vi "GPS.vi"(0 "Data Requested":u16(ring) items=["Time (UTC)"=0, "Status"=1, "Latitude"=2, "Longitude"=4, "Velocity (cm/s)"=6, "Heading (degrees)"=7, "Dist to destination (m)"=8, "Angle to destination (degrees)"=9, "Angle since last req"=10, "Set Destination Latitude"=11, "Set Destination Longitude"=12], 2 "NXT":T1, 3 "Port":T2 items=["Port 1", "Port 2", "Port 3", "Port 4"]) -> (1 "value":i32 format="%.0x", 4 "NXT":T1)   [LabVIEW 2010]
uses:
  <vilib>/NXT/Subs/LVHSConnector.ctl
  <vilib>/NXT/Block Support/NXT_InputPort.ctl
  <vilib>/NXT/Block Support/HWPage.SensorType.ctl
  <vilib>/NXT/Block Support/HWPage.SensorMode.ctl
panel:
  out "Bytes read":u8[](array[numeric]) format="%.0x"
  # "¥ Latitude is represented by an 8-digit integer. If the position is in the northern hemisphere, the number is positive. If the position is in the southern hemisphere, the latitude is negative.\n¥ Longitude is represented by a 9-digit integer. If the position is in the eastern hemisphere, the longitude is positive. If the position is in the western hemisphere, the longitude is negative."
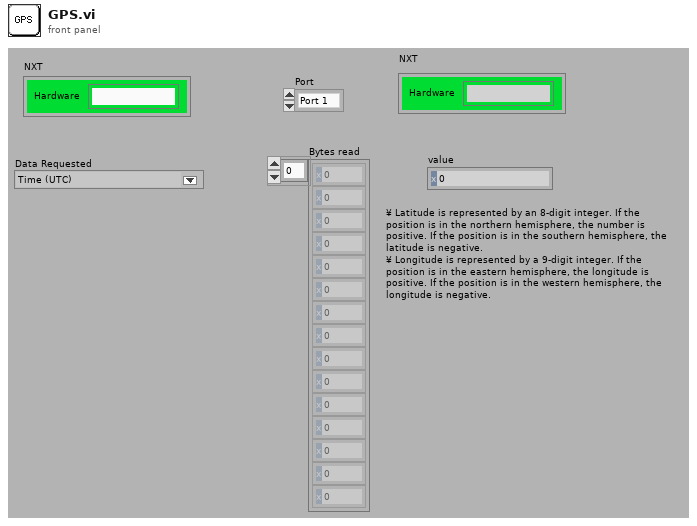
[diagram p1: front panel]
types:
  T1 = typedef "LVHSConnector.ctl" = cluster{"Hardware":string, "Flattened String":string}
  T2 = typedef "NXT_InputPort.ctl" = u8
  T3 = typedef "HWPage.SensorType.ctl" = u8
  T4 = typedef "HWPage.SensorMode.ctl" = u8
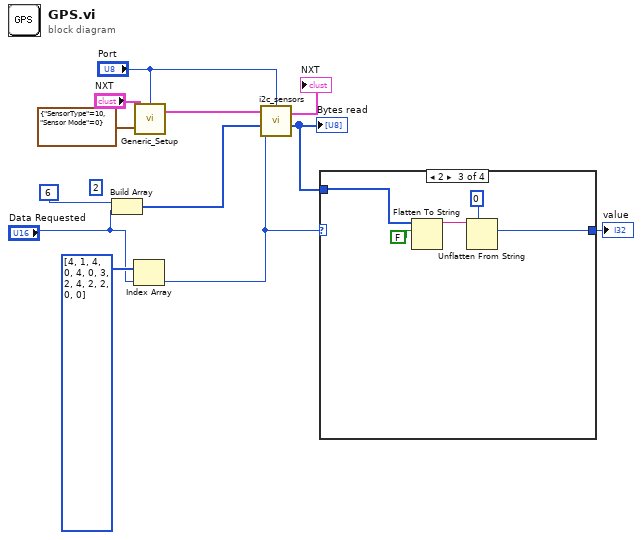
[diagram p0: block diagram]
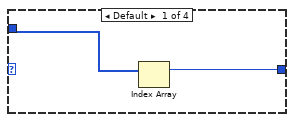
[diagram p2: hidden frame]
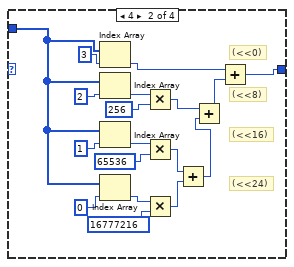
[diagram p3: hidden frame]
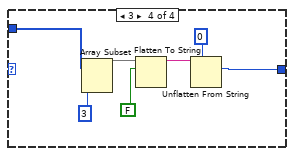
[diagram p4: hidden frame]
diagram:
  (unwired) u8 2 ("Return Length")
  n1 = Build Array(u8 6, "Data Requested") -> (w8:u16[])
  n2 = Index Array(array=u8[] [4, 1, 4, 0, 4, 0, 3, 2, 4, 2, 2, 0, 0], index="Data Requested") -> (element=w1:u8)
  n3 = call <vilib>:"Generic_Setup.vi"("Sensor Setup"=cluster{"SensorType":T3, "Sensor Mode":T4} {"SensorType"=10, "Sensor Mode"=0}, "NXT"="NXT", "Port"="Port") -> ("NXT"=w12:T1)  [unwired: 1 out]
  n4 = call <vilib>:"i2c_sensors.vi"("Return Length"=w1, "Bytes to Write"=w8, "NXT"=w12, "Port"="Port") -> ("Bytes read"=w2:u8[], "NXT"=→"NXT":T1)  [unwired: 1 in, 1 out]
  "Bytes read" <- w2
  n5 = case shown="2" w1 {
    tunnel: w2 -> [w14 w16 w37 w40]
    tunnel: [w13 w15 w34 w41] -> w10
    frame Default {
      n6 = Index Array(array=w14) -> (element=w13:u8)  [unwired: 1 in]
    }
    frame 4 {
      # "(<<24)"
      # "(<<16)"
      # "(<<8)"
      # "(<<0)"
      n7 = Index Array(array=w16, index=3) -> (element=w18:u8)
      n8 = Index Array(array=w16, index=2) -> (element=w25:u8)
      n9 = Index Array(array=w16, index=1) -> (element=w24:u8)
      n10 = Index Array(array=w16, index=0) -> (element=w27:u8)
      n11 = Multiply(x=w25, y=256) -> (x*y=w20:i32)
      n12 = Multiply(x=w24, y=65536) -> (x*y=w22:i32)
      n13 = Multiply(x=w27, y=16777216) -> (x*y=w21:i32)
      n14 = Add(x=w22, y=w21) -> (x+y=w19:i32)
      n15 = Add(x=w20, y=w19) -> (x+y=w17:i32)
      n16 = Add(x=w18, y=w17) -> (x+y=w15:i32)
    }
    frame 2 {
      n17 = Flatten To String(anything=w37, prepend array or string size? (T)=FALSE) -> (data string=w36:string)  [unwired: 2 in, 2 out]
      n18 = Unflatten From String(type=i16 0 ("Return Length"), binary string=w36) -> (value=w34:i16)  [unwired: 3 in, 2 out]
    }
    frame 3 {
      n19 = Array Subset(array=w40, length=3) -> (w39:u8[])  [unwired: 1 in]
      n20 = Flatten To String(anything=w39, prepend array or string size? (T)=FALSE) -> (data string=w44:string)  [unwired: 2 in, 2 out]
      n21 = Unflatten From String(type=0 ("Return Length"), binary string=w44) -> (value=w41:i32)  [unwired: 3 in, 2 out]
    }
  }
  "value" <- w10
